vi "Motion Profiles.vi"() -> ()   [LabVIEW 2019]
uses:
  <vilib>/Rock Robotics/WPI/ThirdParty/Phoenix-LabVIEW/Motor Controller/Controls/CTRE_Phoenix_MotorControl_BufferedTrajectoryPointStream_DeviceRef.ctl
panel:
  in  "MP_CUSTOM":cluster{"MP_left":T1, "MP_right":T1}
  in  "MP_RIGHT":cluster{"MP_left":T1, "MP_right":T1}
  in  "MP_CENTER":cluster{"MP_left":T1, "MP_right":T1}
  in  "MP_LEFT":cluster{"MP_left":T1, "MP_right":T1}
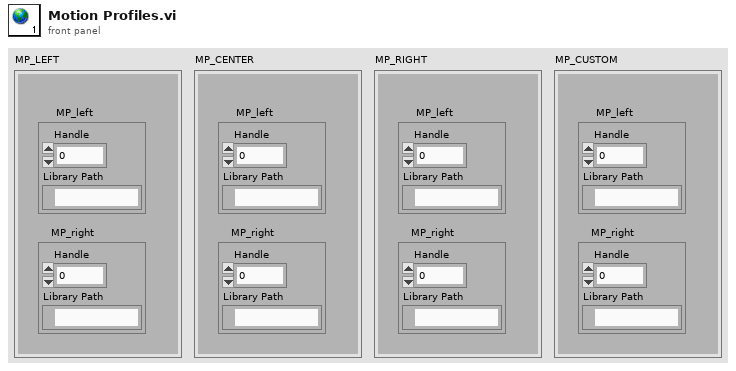
[diagram p1: front panel]
types:
  T1 = typedef "CTRE_Phoenix_MotorControl_BufferedTrajectoryPointStream_DeviceRef.ctl" = cluster{"Handle":u64, "Library Path":path}
diagram:
